vi "SVT Sound Level (N Ch).vi"(0 "scaled signals [EU]":waveform(dbl)[](array[waveform]), 1 "integration time [s]":dbl=1.0 format="%.2f", 5 "measurement selection":T1={"Leq"=TRUE, "Running Leq"=FALSE, "Exponential"=FALSE, "Peak"=FALSE}, 7 "exponential mode":enum16{"Slow", "Fast", "Impulse", "Custom"}(ring)=enum."Fast", 9 "time constant [ms]":dbl=125.0 format="%.2f", 11 "error in (no error)":errorcluster, 12 "restart averaging (F)":bool) -> (3 "exp avg sound levels [dB EU]":waveform(dbl)[](array[waveform]), 4 "Leq sound levels [dB EU]":waveform(dbl)[](array[waveform]), 6 "running Leq sound levels [dB EU]":waveform(dbl)[](array[waveform]), 8 "peak sound levels [dB pk EU]":waveform(dbl)[](array[waveform]), 14 "unit labels":string[](array[string]), 15 "error out":errorcluster)   [LabVIEW 2017, in "SoundVib_SoundLevel.lvlib"]
doc: "Computes several sound level measurements including equivalent continuous level (Leq), running Leq sound levels, exponential averaged sound level, and the peak sound level. Wire data to the <B>scaled signal [EU]</B> input to determine the polymorphic instance to use or manually select the instance."
uses:
  <vilib>/addons/Sound and Vibration/svt_Level/SoundVib_SoundLevel.lvlib
  <vilib>/addons/Sound and Vibration/svt_Level/SVL Peak Sound Level (N Ch).vi
  <vilib>/addons/Sound and Vibration/svt_Level/SVL Decimated Exp Avg Sound Level (N Ch).vi
  <vilib>/addons/Sound and Vibration/svt_Level/SVL Running Leq Sound Level (N Ch).vi
  <vilib>/addons/Sound and Vibration/svt_Level/SVL Leq Sound Level (N Ch).vi
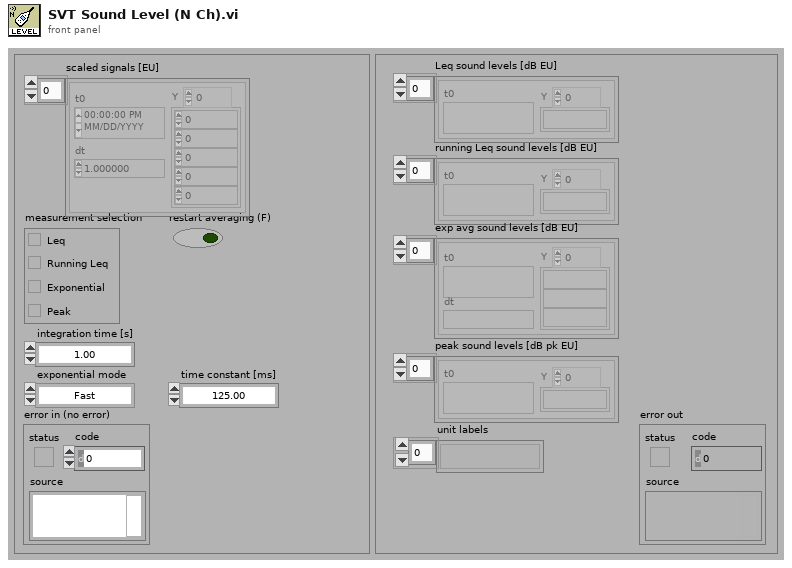
[diagram p1: front panel]
types:
  T1 = cluster{"Leq":bool, "Running Leq":bool, "Exponential":bool, "Peak":bool}
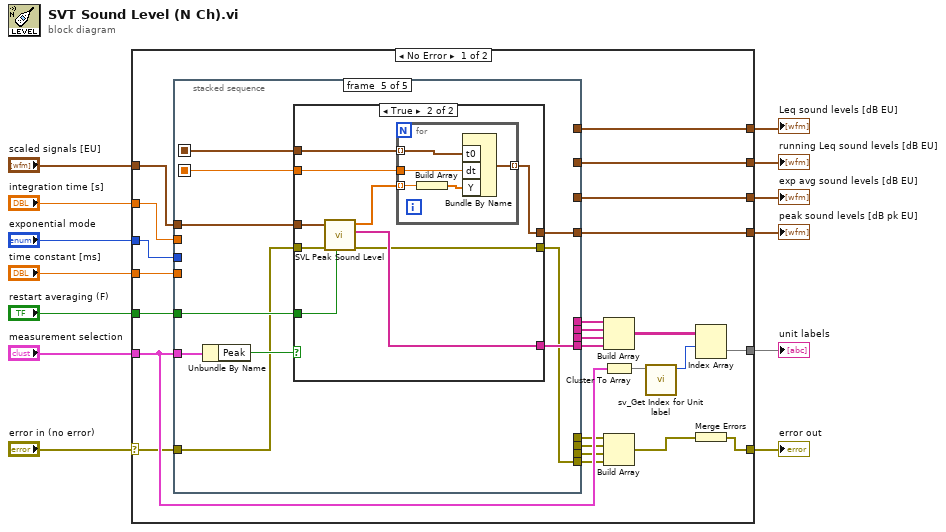
[diagram p0: block diagram]
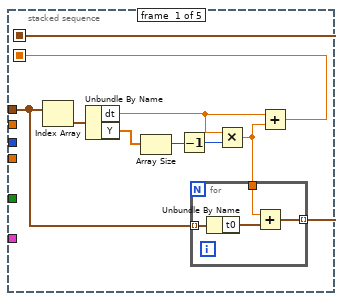
[diagram p2: hidden frame]
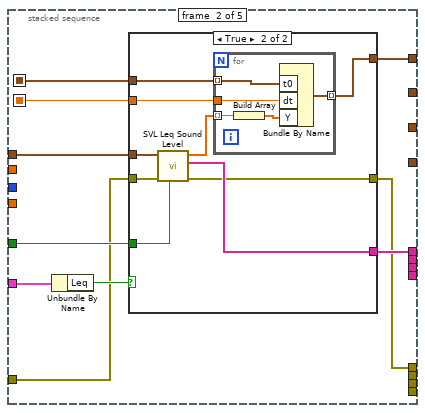
[diagram p3: hidden frame]
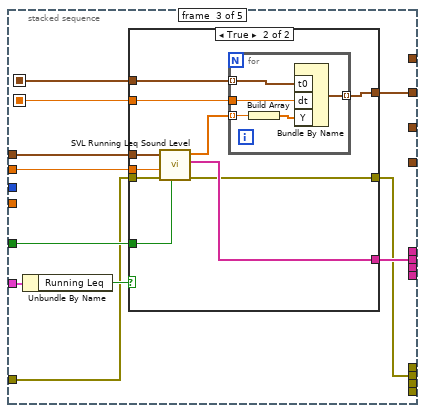
[diagram p5: hidden frame]
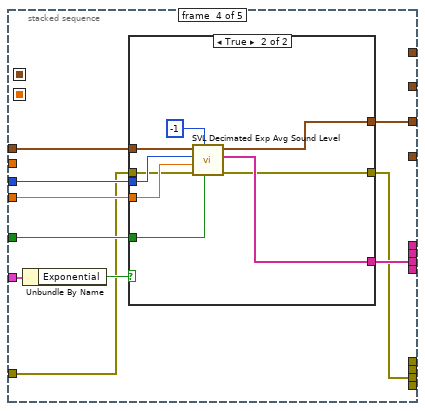
[diagram p7: hidden frame]
diagram:
  n1 = case shown="No Error" "error in (no error)" {
    selector: "error in (no error)" -> [w18 w149]
    tunnel: "scaled signals [EU]" -> [w38 _]
    tunnel: "restart averaging (F)" -> [w37 _]
    tunnel: [w36 _] -> w4
    tunnel: [w35 _] -> w3
    tunnel: "integration time [s]" -> [w34 _]
    tunnel: "exponential mode" -> [w33 _]
    tunnel: "time constant [ms]" -> [w32 _]
    tunnel: [w31 _] -> w2
    tunnel: [w30 _] -> w1
    tunnel: "measurement selection" -> [w29 _]
    tunnel: [w14 _] -> w8
    tunnel: [w19 w149] -> w7
    frame No Error {
      n2 = stacked-sequence {
        seq-local: [w44 _ _ _ _] -> [_ w56 w82 _ w128]
        seq-local: [w43 _ _ _ _] -> [_ w57 w83 _ w129]
        tunnel: w29 -> [_ w61 w87 w113 w133]
        tunnel: w38 -> [w42 w59 w85 w111 w131]
        tunnel: w37 -> [_ w58 w84 w110 w130]
        tunnel: [_ w55 _ _ _] -> w36
        tunnel: [_ _ w81 _ _] -> w35
        tunnel: w34 -> [_ _ w80 _ _]
        tunnel: w33 -> [_ _ _ w109 _]
        tunnel: w32 -> [_ _ _ w108 _]
        tunnel: [_ _ _ w107 _] -> w31
        tunnel: [_ _ _ _ w127] -> w30
        tunnel: [_ w54 _ _ _] -> w28
        tunnel: [_ _ w79 _ _] -> w27
        tunnel: [_ _ _ w106 _] -> w26
        tunnel: [_ _ _ _ w126] -> w25
        tunnel: w18 -> [_ w53 w78 w105 w125]
        tunnel: [_ w52 _ _ _] -> w24
        tunnel: [_ _ w77 _ _] -> w23
        tunnel: [_ _ _ w104 _] -> w22
        tunnel: [_ _ _ _ w124] -> w21
        frame #0 {
          n3 = Index Array(array=w42) -> (element=w41:waveform(dbl))  [unwired: 1 in]
          n4 = Unbundle By Name(w41) -> ("dt"=w39:dbl, "Y"=w47:dbl[])
          n5 = Array Size(array=w47) -> (size(s)=w46:i32)
          n6 = Decrement(x=w46) -> (x-1=w45:i32)
          n7 = Multiply(x=w39, y=w45) -> (x*y=w40:dbl)
          n8 = for {
            tunnel: w42 -> [w51] mode=indexing
            tunnel: w40 -> [w50]
            tunnel: [w48] -> w43 mode=indexing
            n9 = Unbundle By Name(w51) -> ("t0"=w49:timestamp)
            n10 = Add(x=w50, y=w49) -> (x+y=w48:timestamp)
          }
          n11 = Add(x=w39, y=w40) -> (x+y=w44:dbl)
        }
        frame #1 {
          n12 = Unbundle By Name(w61) -> ("Leq"=w60:bool)
          n13 = case shown="True" w60 {
            tunnel: w59 -> [_ w71]
            tunnel: w58 -> [_ w70]
            tunnel: w57 -> [_ w69]
            tunnel: w56 -> [_ w68]
            tunnel: [_ w67] -> w55
            tunnel: [_ w66] -> w54
            tunnel: w53 -> [w62 w65]
            tunnel: [w62 w64] -> w52
            frame False {
            }
            frame True {
              n14 = call-poly <vilib>:"SVL Leq Sound Level.vi"("restart averaging (F)"=w70, "error in (no error)"=w65, "scaled signals [EU]"=w71) -> ("error out"=w64:errorcluster, "unit labels"=w66:string[], "Leq sound levels [dB EU]"=w63:dbl[])  [unwired: 6 in]
              n15 = for {
                tunnel: w69 -> [w76] mode=indexing
                tunnel: w68 -> [w75]
                tunnel: [w74] -> w67 mode=indexing
                tunnel: w63 -> [w73] mode=indexing
                n16 = Build Array(w73) -> (w72:dbl[])
                n17 = Bundle By Name("t0"=w76, "dt"=w75, "Y"=w72) -> (w74:waveform(dbl))  [unwired: 1 in]
              }
            }
          }
        }
        frame #2 {
          n18 = Unbundle By Name(w87) -> ("Running Leq"=w86:bool)
          n19 = case shown="True" w86 {
            tunnel: w85 -> [_ w98]
            tunnel: w84 -> [_ w97]
            tunnel: w83 -> [_ w89]
            tunnel: w82 -> [_ w90]
            tunnel: [_ w92] -> w81
            tunnel: w80 -> [_ w96]
            tunnel: [_ w95] -> w79
            tunnel: w78 -> [w88 w94]
            tunnel: [w88 w93] -> w77
            frame False {
            }
            frame True {
              n20 = call-poly <vilib>:"SVL Running Leq Sound Level.vi"("restart averaging (F)"=w97, "error in (no error)"=w94, "integration time [s]"=w96, "scaled signals [EU]"=w98) -> ("error out"=w93:errorcluster, "unit labels"=w95:string[], "running Leq sound levels [dB EU]"=w91:dbl[])  [unwired: 4 in, 1 out]
              n21 = for {
                tunnel: w89 -> [w103] mode=indexing
                tunnel: w90 -> [w102]
                tunnel: [w101] -> w92 mode=indexing
                tunnel: w91 -> [w100] mode=indexing
                n22 = Build Array(w100) -> (w99:dbl[])
                n23 = Bundle By Name("t0"=w103, "dt"=w102, "Y"=w99) -> (w101:waveform(dbl))  [unwired: 1 in]
              }
            }
          }
        }
        frame #3 {
          n24 = Unbundle By Name(w113) -> ("Exponential"=w112:bool)
          n25 = case shown="True" w112 {
            tunnel: w111 -> [_ w123]
            tunnel: w110 -> [_ w122]
            tunnel: w109 -> [_ w121]
            tunnel: w108 -> [_ w120]
            tunnel: [_ w118] -> w107
            tunnel: [_ w117] -> w106
            tunnel: w105 -> [w114 w116]
            tunnel: [w114 w115] -> w104
            frame False {
            }
            frame True {
              n26 = call-poly <vilib>:"SVL Decimated Exp Avg Sound Level.vi"("restart averaging (F)"=w122, "decimation factor"=-1, "error in (no error)"=w116, "time constant [ms]"=w120, "exponential mode"=w121, "scaled signals [EU]"=w123) -> ("error out"=w115:errorcluster, "unit labels"=w117:string[], "decimated exp avg sound levels [dB EU]"=w118:waveform(dbl)[])  [unwired: 1 in, 2 out]
            }
          }
        }
        frame #4 {
          n27 = Unbundle By Name(w133) -> ("Peak"=w132:bool)
          n28 = case shown="True" w132 {
            tunnel: w131 -> [_ w143]
            tunnel: w130 -> [_ w142]
            tunnel: w129 -> [_ w136]
            tunnel: w128 -> [_ w138]
            tunnel: [_ w135] -> w127
            tunnel: [_ w141] -> w126
            tunnel: w125 -> [w134 w140]
            tunnel: [w134 w139] -> w124
            frame False {
            }
            frame True {
              n29 = call-poly <vilib>:"SVL Peak Sound Level.vi"("restart averaging (F)"=w142, "error in (no error)"=w140, "scaled signals [EU]"=w143) -> ("error out"=w139:errorcluster, "unit labels"=w141:string[], "peak sound levels [dB pk EU]"=w137:dbl[])  [unwired: 6 in]
              n30 = for {
                tunnel: w136 -> [w148] mode=indexing
                tunnel: w138 -> [w147]
                tunnel: [w146] -> w135 mode=indexing
                tunnel: w137 -> [w145] mode=indexing
                n31 = Build Array(w145) -> (w144:dbl[])
                n32 = Bundle By Name("t0"=w148, "dt"=w147, "Y"=w144) -> (w146:waveform(dbl))  [unwired: 1 in]
              }
            }
          }
        }
      }
      n33 = Build Array(w28, w27, w26, w25) -> (w16:string[][])
      n34 = Cluster To Array(cluster=w29) -> (array=w17:bool[])
      n35 = Build Array(w24, w23, w22, w21) -> (w20:errorcluster[])
      n36 = call <vilib>:"sv_Get Index for Unit label.vi"("measurement selection"=w17) -> ("index"=w15:i32)  [unwired: 10 in]
      n37 = Index Array(array=w16, index (row)=w15) -> (element=w14:string[])  [unwired: 1 in]
      n38 = Merge Errors(w20) -> (w19:errorcluster)
    }
    frame Error {
    }
  }
  "error out" <- w7
  "unit labels" <- w8
  "peak sound levels [dB pk EU]" <- w1
  "exp avg sound levels [dB EU]" <- w2
  "Leq sound levels [dB EU]" <- w4
  "running Leq sound levels [dB EU]" <- w3
